vi "Convex Hull_Low Hull.vi"(11 "Points":cluster{"x":dbl, "y":dbl, "index":i32}[](array[cluster])) -> (3 "Low Hull":cluster{"x":dbl, "y":dbl, "index":i32}[](array[cluster]))   [LabVIEW 2017, in "NI_AAL_Geometry.lvlib"]
uses:
  <vilib>/Analysis/NI_AAL_Geometry.lvlib
  <vilib>/Analysis/geometry.llb/Triangle Area.vi
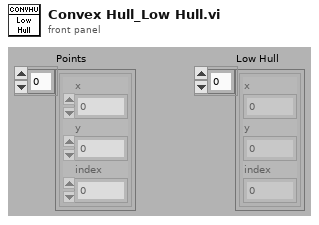
[diagram p1: front panel]
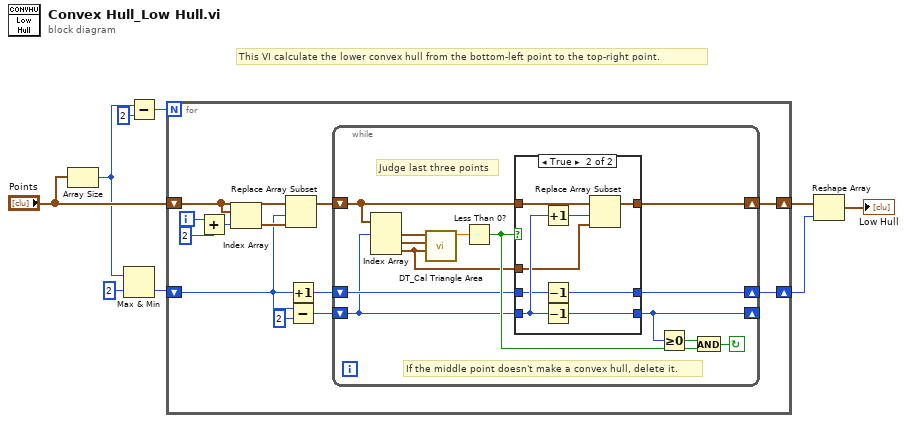
[diagram p0: block diagram]
diagram:
  # "This VI calculate the lower convex hull from the bottom-left point to the top-right point."
  n1 = Array Size(array="Points") -> (size(s)=w1:i32)
  n2 = Max & Min(x=w1, y=2) -> (min(x,y)=w3:i32)  [unwired: 1 out]
  n3 = Subtract(x=w1, y=2) -> (x-y=w8:i32)
  n4 = for {
    N: w8 -> [_]
    shift-right: [w21] -> w6
    shift-left: "Points" -> [w19]
    shift-right: [w13] -> w5
    shift-left: w3 -> [w11]
    i -> [w17]
    n5 = Add(x=w17, y=2) -> (x+y=w15:i32)
    n6 = Index Array(array=w19, index=w15) -> (element=w18:cluster{"x":dbl, "y":dbl, "index":i32})
    n7 = Replace Array Subset(array=w19, new element=w18, index=w11) -> (w20:cluster{"x":dbl, "y":dbl, "index":i32}[])
    n8 = Increment(x=w11) -> (x+1=w14:i32)
    n9 = Subtract(x=w11, y=2) -> (x-y=w10:i32)
    n10 = while {
      shift-right: [w31] -> w21
      shift-left: w20 -> [w33]
      shift-right: [w25] -> w13
      shift-left: w14 -> [w24]
      shift-right: [w22] -> _
      shift-left: w10 -> [w23]
      stop <- w32 continue-if-true
      # "If the middle point doesn't make a convex hull, delete it."
      # "Judge last three points"
      n11 = Index Array(array=w33, index #1=w23) -> (element #1=w28:cluster{"x":dbl, "y":dbl, "index":i32}, element #2=w27:cluster{"x":dbl, "y":dbl, "index":i32}, element #3=w26:cluster{"x":dbl, "y":dbl, "index":i32})  [unwired: 2 in]
      n12 = call <vilib>:"DT_Cal Triangle Area.vi"("p 3"=w26, "p 2"=w27, "p 1"=w28) -> ("area"=w34:dbl)  [unwired: 8 in]
      n13 = Less Than 0?(x=w34) -> (x < 0?=w30:bool)
      n14 = case shown="True" w30 {
        tunnel: w33 -> [w37 w45]
        tunnel: [w37 w43] -> w31
        tunnel: w23 -> [w35 w42]
        tunnel: [w35 w41] -> w22
        tunnel: w26 -> [_ w40]
        tunnel: [w36 w39] -> w25
        tunnel: w24 -> [w36 w38]
        frame False {
        }
        frame True {
          n15 = Increment(x=w42) -> (x+1=w44:i32)
          n16 = Decrement(x=w38) -> (x-1=w39:i32)
          n17 = Decrement(x=w42) -> (x-1=w41:i32)
          n18 = Replace Array Subset(array=w45, new element=w40, index=w44) -> (w43:cluster{"x":dbl, "y":dbl, "index":i32}[])
        }
      }
      n19 = Greater Or Equal To 0?(x=w22) -> (x >= 0?=w29:bool)
      n20 = And(x=w29, y=w30) -> (x .and. y?=w32:bool)
    }
  }
  n21 = Reshape Array(w6, w5) -> (→"Low Hull":cluster{"x":dbl, "y":dbl, "index":i32}[])
